vi "Tiepie-takeData-2018-04-26.vi"(2 "error in (no error)":errorcluster, 4 "ADC parameter":T1, 5 "Laser parameter":T3) -> (0 "error out":errorcluster, 1 "output cluster":cluster{i32[], dbl[]})   [LabVIEW 2013]
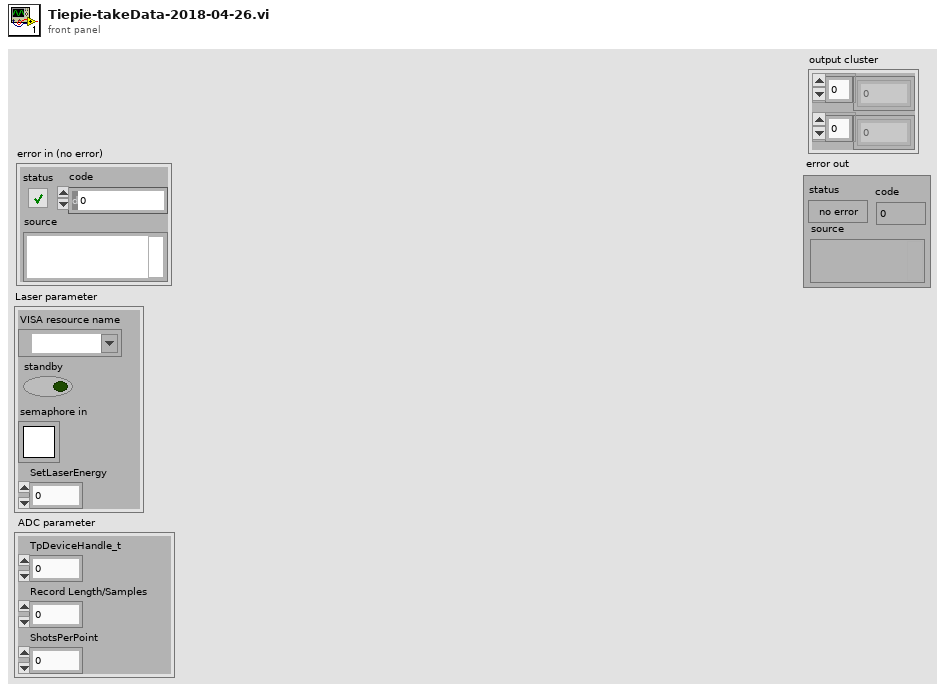
[diagram p1: front panel]
types:
  T1 = cluster{"TpDeviceHandle_t":u32, "Record Length/Samples":u64, "ShotsPerPoint":u16}
  T2 = typedef "Semaphore RefNum" = refnum<k1>
  T3 = cluster{"VISA resource name":refnum<visa-resource-name>, "standby":bool, "semaphore in":T2, "SetLaserEnergy":dbl}
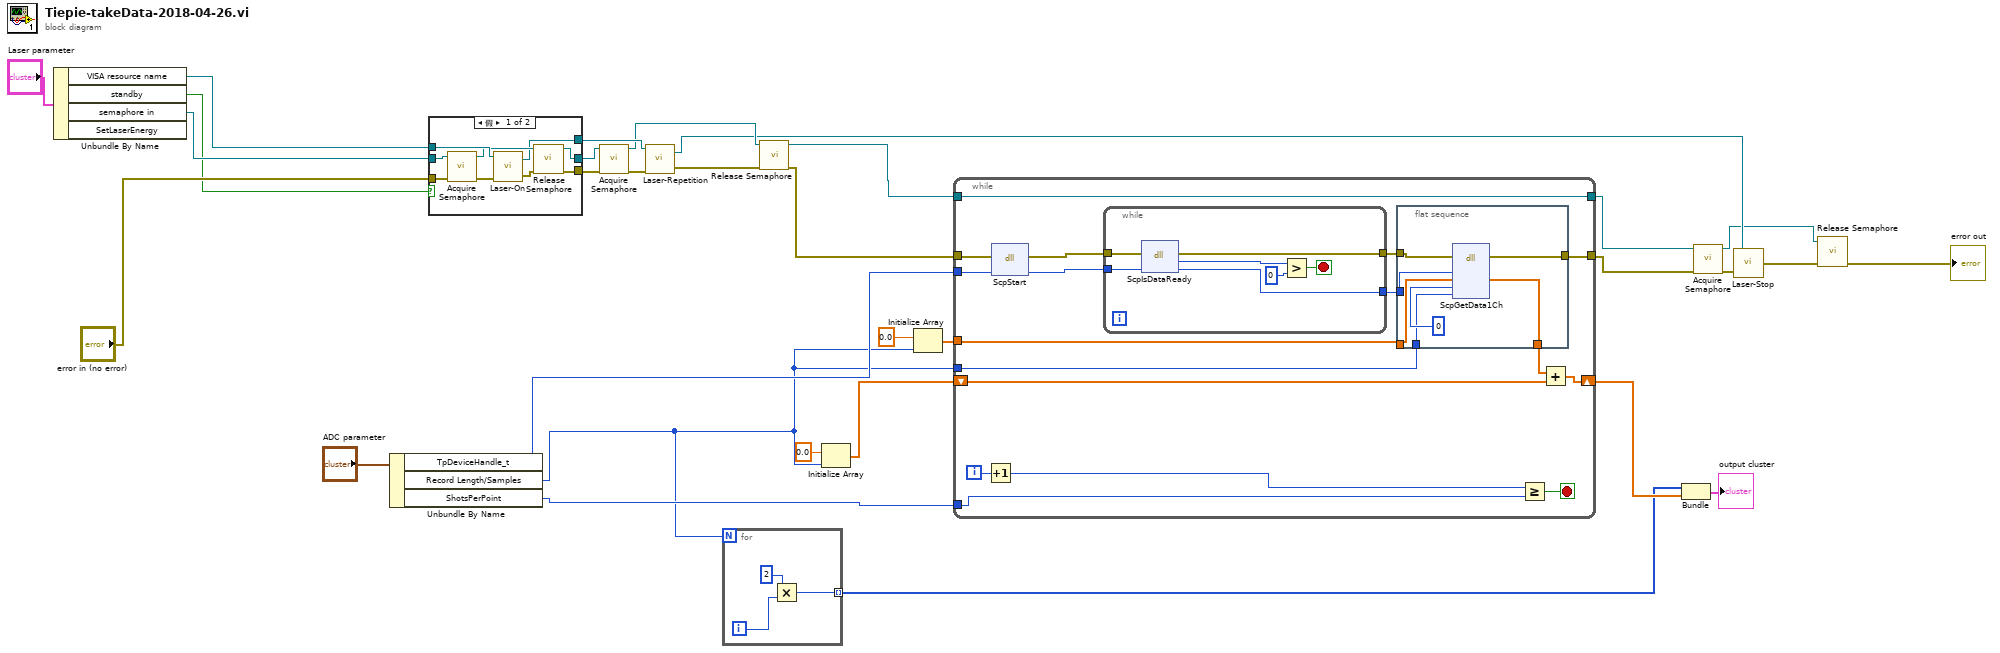
[diagram p0: block diagram]
diagram:
  n1 = Unbundle By Name("Laser parameter") -> ("VISA resource name"=w15:refnum<visa-resource-name>, "standby"=w14:bool, "semaphore in"=w25:T2)  [unwired: 1 out]
  n2 = Unbundle By Name("ADC parameter") -> ("TpDeviceHandle_t"=w23:u32, "Record Length/Samples"=w19:u64, "ShotsPerPoint"=w22:u16)
  n3 = case shown="假" w14 {
    tunnel: "error in (no error)" -> [w40 w41]
    tunnel: w25 -> [w39 w42]
    tunnel: w15 -> [w36 w43]
    tunnel: [w34 w41] -> w12
    tunnel: [w33 w42] -> w13
    tunnel: [w32 w43] -> w11
    frame False {
      n4 = call <vilib>:"Acquire Semaphore.vi"("error in (no error)"=w40, "semaphore"=w39) -> ("error out"=w38:errorcluster, "semaphore out"=w35:T2)  [unwired: 3 in, 1 out]
      n5 = call "Laser-On.vi"("error in (no error)"=w38, "VISA resource name"=w36) -> ("error out"=w37:errorcluster, "VISA resource name out"=w32:refnum<visa-resource-name>)  [unwired: 2 in]
      n6 = call <vilib>:"Release Semaphore.vi"("error in (no error)"=w37, "semaphore"=w35) -> ("error out"=w34:errorcluster, "semaphore out"=w33:T2)  [unwired: 4 in]
    }
    frame True {
    }
  }
  n7 = call <vilib>:"Acquire Semaphore.vi"("error in (no error)"=w12, "semaphore"=w13) -> ("error out"=w10:errorcluster, "semaphore out"=w8:T2)  [unwired: 3 in, 1 out]
  n8 = call "Laser-Repetition.vi"("error in (no error)"=w10, "VISA resource name"=w11) -> ("error out"=w9:errorcluster, "VISA resource name out"=w7:refnum<visa-resource-name>)  [unwired: 2 in]
  n9 = for {
    N: w19 -> [_]
    tunnel: [w44] -> w17 mode=indexing
    i -> [w46]
    n10 = Multiply(x=2, y=w46) -> (x*y=w44:i32)
  }
  n11 = call <vilib>:"Release Semaphore.vi"("error in (no error)"=w9, "semaphore"=w8) -> ("error out"=w6:errorcluster, "semaphore out"=w2:T2)  [unwired: 4 in]
  n12 = Initialize Array(0.0 ("element"), w19) -> (w30:dbl[])
  n13 = Initialize Array(0.0, w19) -> (w28:dbl[])
  n14 = while {
    tunnel: w23 -> [w63]
    shift-right: [w58] -> w18
    shift-left: w30 -> [w59]
    tunnel: w19 -> [w52]
    tunnel: w28 -> [w51]
    tunnel: w22 -> [w50]
    tunnel: [w49] -> w5
    tunnel: w6 -> [w48]
    tunnel: w2 -> [w47]
    tunnel: [w47] -> w1
    i -> [w57]
    stop <- w53 stop-if-true
    n15 = Increment(x=w57) -> (x+1=w56:i32)
    n16 = dll-call lib="PTH1Tabs CUsers82158Desktop上海项目TOF software\t数据卡\nlibtiepie.dll" fn="ScpStart"(error in=w48, "TpDeviceHandle_t"=w63) -> (error out=w62:errorcluster, "TpDeviceHandle_t"=w61:u32)  [unwired: 3 in, 1 out]
    n17 = while {
      tunnel: w62 -> [w77]
      tunnel: w61 -> [w76]
      tunnel: [w75] -> w55
      tunnel: [w74] -> w54
      stop <- w71 stop-if-true
      n18 = dll-call lib="PTH1Tabs CUsers82158Desktop上海项目TOF software\t数据卡\nlibtiepie.dll" fn="ScpIsDataReady"(error in=w77, "TpDeviceHandle_t"=w76) -> (error out=w75:errorcluster, "DataReady"=w72:u8, "TpDeviceHandle_t"=w74:u32)  [unwired: 2 in, 1 out]
      n19 = Greater?(x=w72, y=0 ("index")) -> (0:w71:bool)
    }
    n20 = flat-sequence {
      tunnel: [w70] -> w60
      tunnel: w55 -> [w69]
      tunnel: w54 -> [w68]
      tunnel: w52 -> [w66]
      tunnel: w51 -> [w65]
      tunnel: [w64] -> w49
      frame #0 {
        n21 = dll-call lib="PTH1Tabs CUsers82158Desktop上海项目TOF software\t数据卡\nlibtiepie.dll" fn="ScpGetData1Ch"(error in=w69, "TpDeviceHandle_t"=w68, "pBufferCh1"=w65, "qwStartIndex"=u64 0, "qwSampleCount"=w66) -> (error out=w64:errorcluster, "pBufferCh1"=w70:sgl[])  [unwired: 6 in, 1 out]
      }
    }
    n22 = Greater Or Equal?(x=w56, y=w50) -> (x >= y?=w53:bool)
    n23 = Add(x=w60, y=w59) -> (x+y=w58:dbl[])
  }
  n24 = Bundle(w17, w18) -> (→"output cluster":cluster{i32[], dbl[]})  [unwired: 1 in]
  n25 = call <vilib>:"Acquire Semaphore.vi"("error in (no error)"=w5, "semaphore"=w1) -> ("error out"=w4:errorcluster, "semaphore out"=w3:T2)  [unwired: 3 in, 1 out]
  n26 = call "Laser-Stop.vi"("error in (no error)"=w4, "VISA resource name"=w7) -> ("error out"=w20:errorcluster)
  n27 = call <vilib>:"Release Semaphore.vi"("error in (no error)"=w20, "semaphore"=w3) -> ("error out"=→"error out":errorcluster)  [unwired: 4 in, 1 out]
